vi "Get Device Info.vi"(11 "EDS in":refnum<class "EDS.lvclass">) -> (2 "Device Info":refnum<class "Device Info.lvclass">, 3 "EDS out":refnum<class "EDS.lvclass">)   [LabVIEW 2024, in "EDS.lvlib" / "EDS.lvclass"]
uses:
  EDS.lvclass
  EDS.lvclass/EDS.ctl
  Device Info/Device Info.lvclass
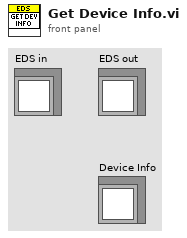
[diagram p1: front panel]
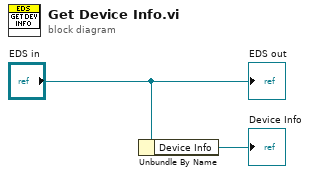
[diagram p0: block diagram]
diagram:
  n1 = Unbundle By Name("EDS in") -> ("Device Info"=→"Device Info":refnum<class "Device Info.lvclass">)
  "EDS out" <- "EDS in"
